vi "1midterm.vi"() -> ()   [LabVIEW 2024]
uses:
  <userlib>/SerialVIs/subs/portX.xctl
panel:
  in  "File Path 5":path=path "C:/Users/mbyjo/Downloads/tish---success!-made-with-Voicemod.wav"
  in  "File Path 4":path=path "C:/Users/mbyjo/Downloads/eye-of-the-tiger-intro-made-with-Voicemod.wav"
  in  "File Path 3":path=path "C:/Users/mbyjo/Downloads/game-over-made-with-Voicemod.wav"
  in  "File Path 2":path=path "C:/Users/mbyjo/Downloads/evil-laugh-made-with-Voicemod.wav"
  in  "File Path":path=path "C:/Users/mbyjo/Downloads/saw-do-you-wanna-play-a-game_-made-with-Voicemod.wav"
  out "Arm Range 2":cluster{"X":dbl, "Y":dbl}[](graph)
  out "Angle 3":dbl
  out "Angle 2":dbl
  out "Angle1":dbl
  out "Arm Range 1":picture
  out "Robot arm Final Position":cluster{"x2":dbl, "y2":dbl}
  out "2D Simulation of Robot Arm":picture
  out "Angles(q)":dbl[](array[numeric])
  in  "Arm Lengths":cluster{"L 1":dbl, "L 2":dbl, "L4":dbl}
  in  "portX":refnum<visa-resource-name>(xcontrol)
  # "DO YOU WANNA PLAY A GAME?"
  # "PRESS THE ARROW TO GET STARTED!"
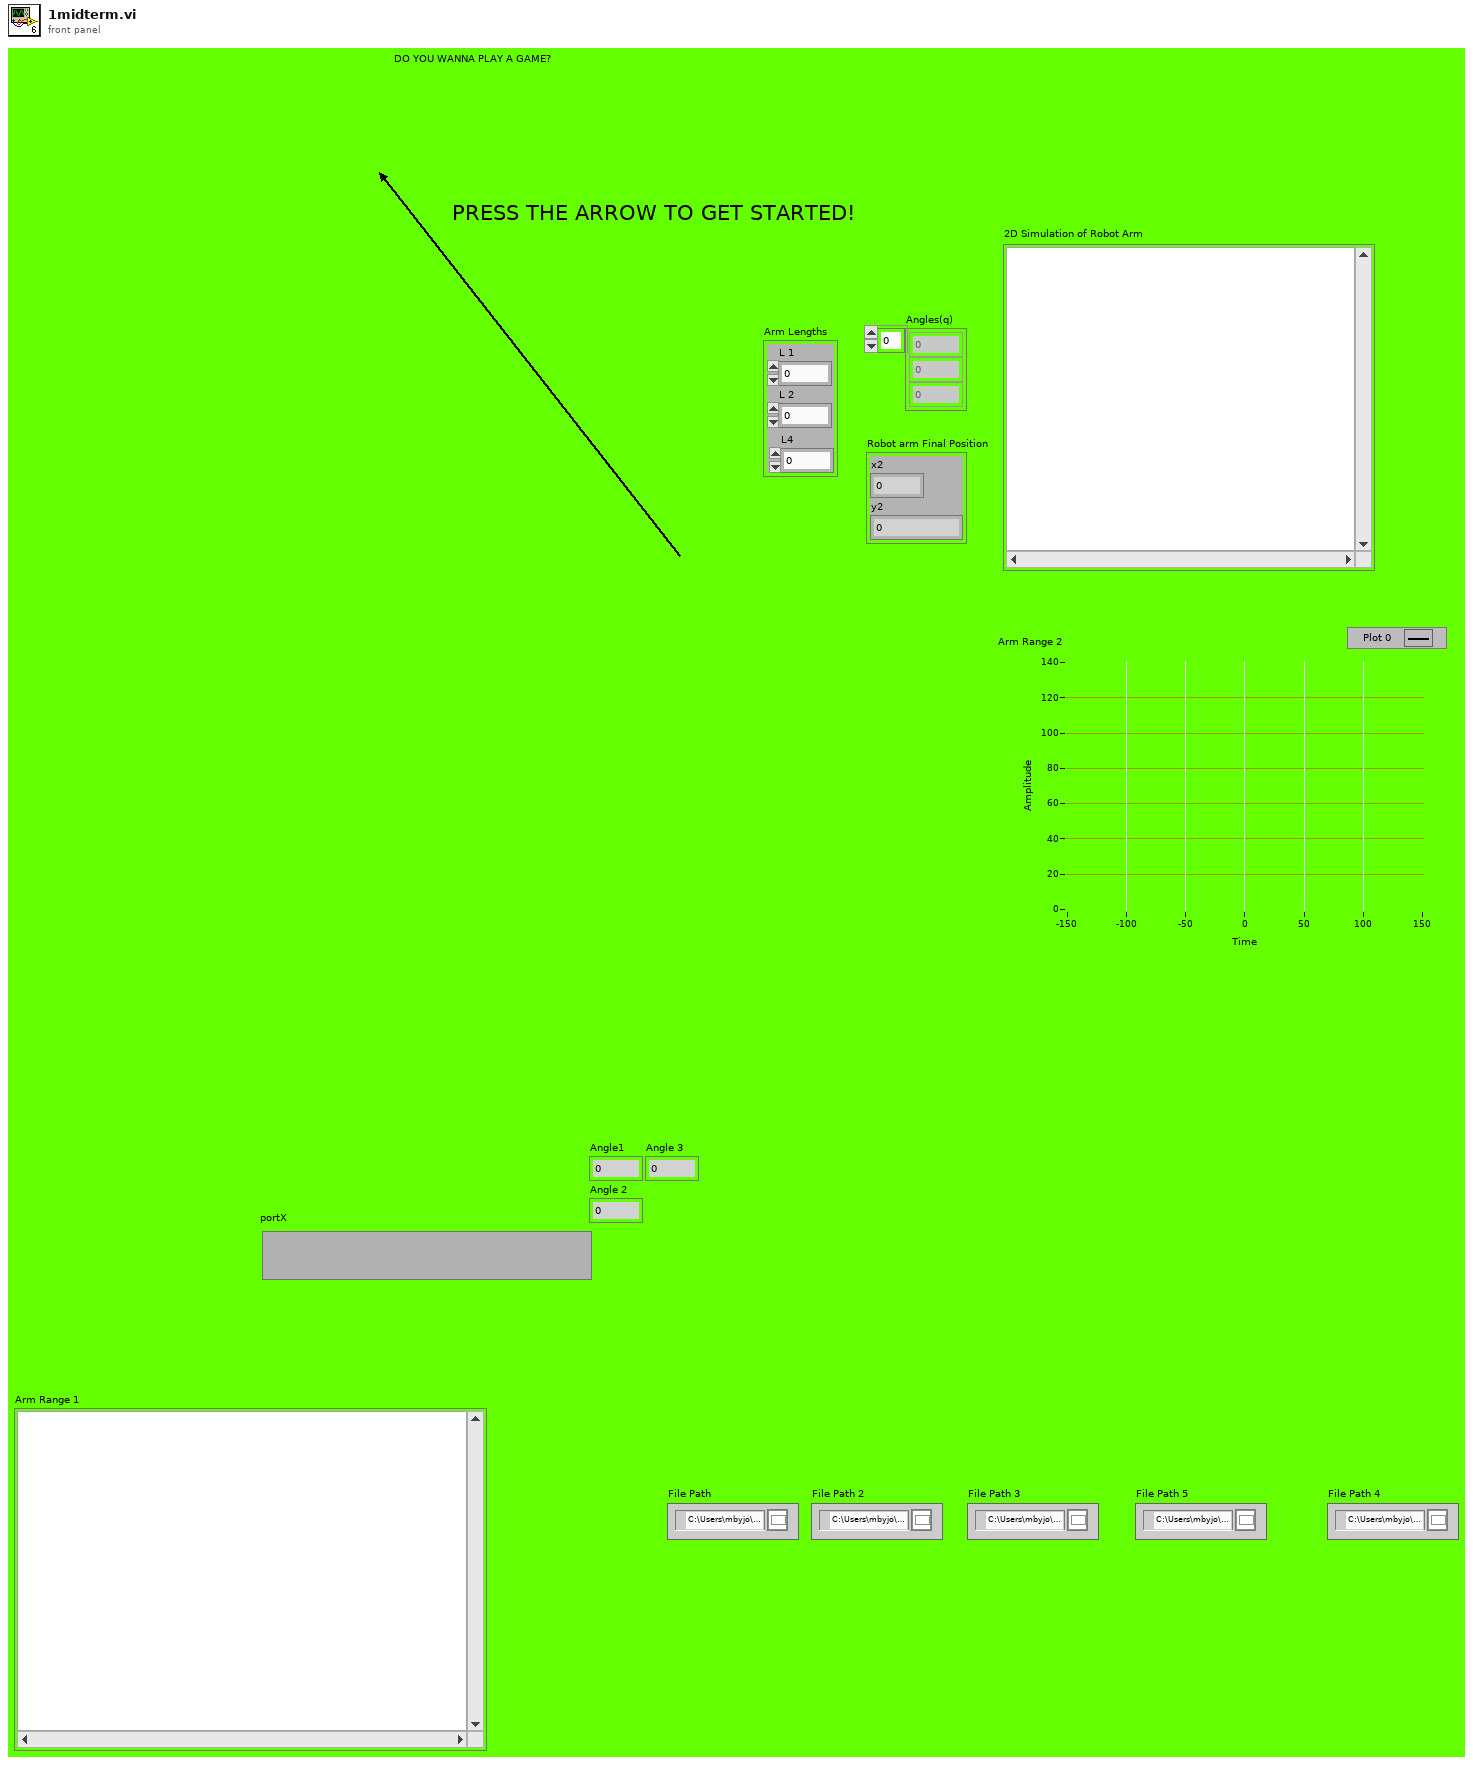
[diagram p1: front panel]
types:
  T1 = cluster{"Width":u16, "Style":enum32{"Solid", "Dash", "Dot", "DashDot", "DashDotDot"}}
  T2 = cluster{"Angles(q)[0]":dbl, "Angles(q)[1]":dbl, "Angles(q)[2]":dbl, "Angles(q)[3]":dbl, "Angles(q)[4]":dbl, "Angles(q)[5]":dbl, "Angles(q)[6]":dbl, "Angles(q)[7]":dbl, "Angles(q)[8]":dbl}
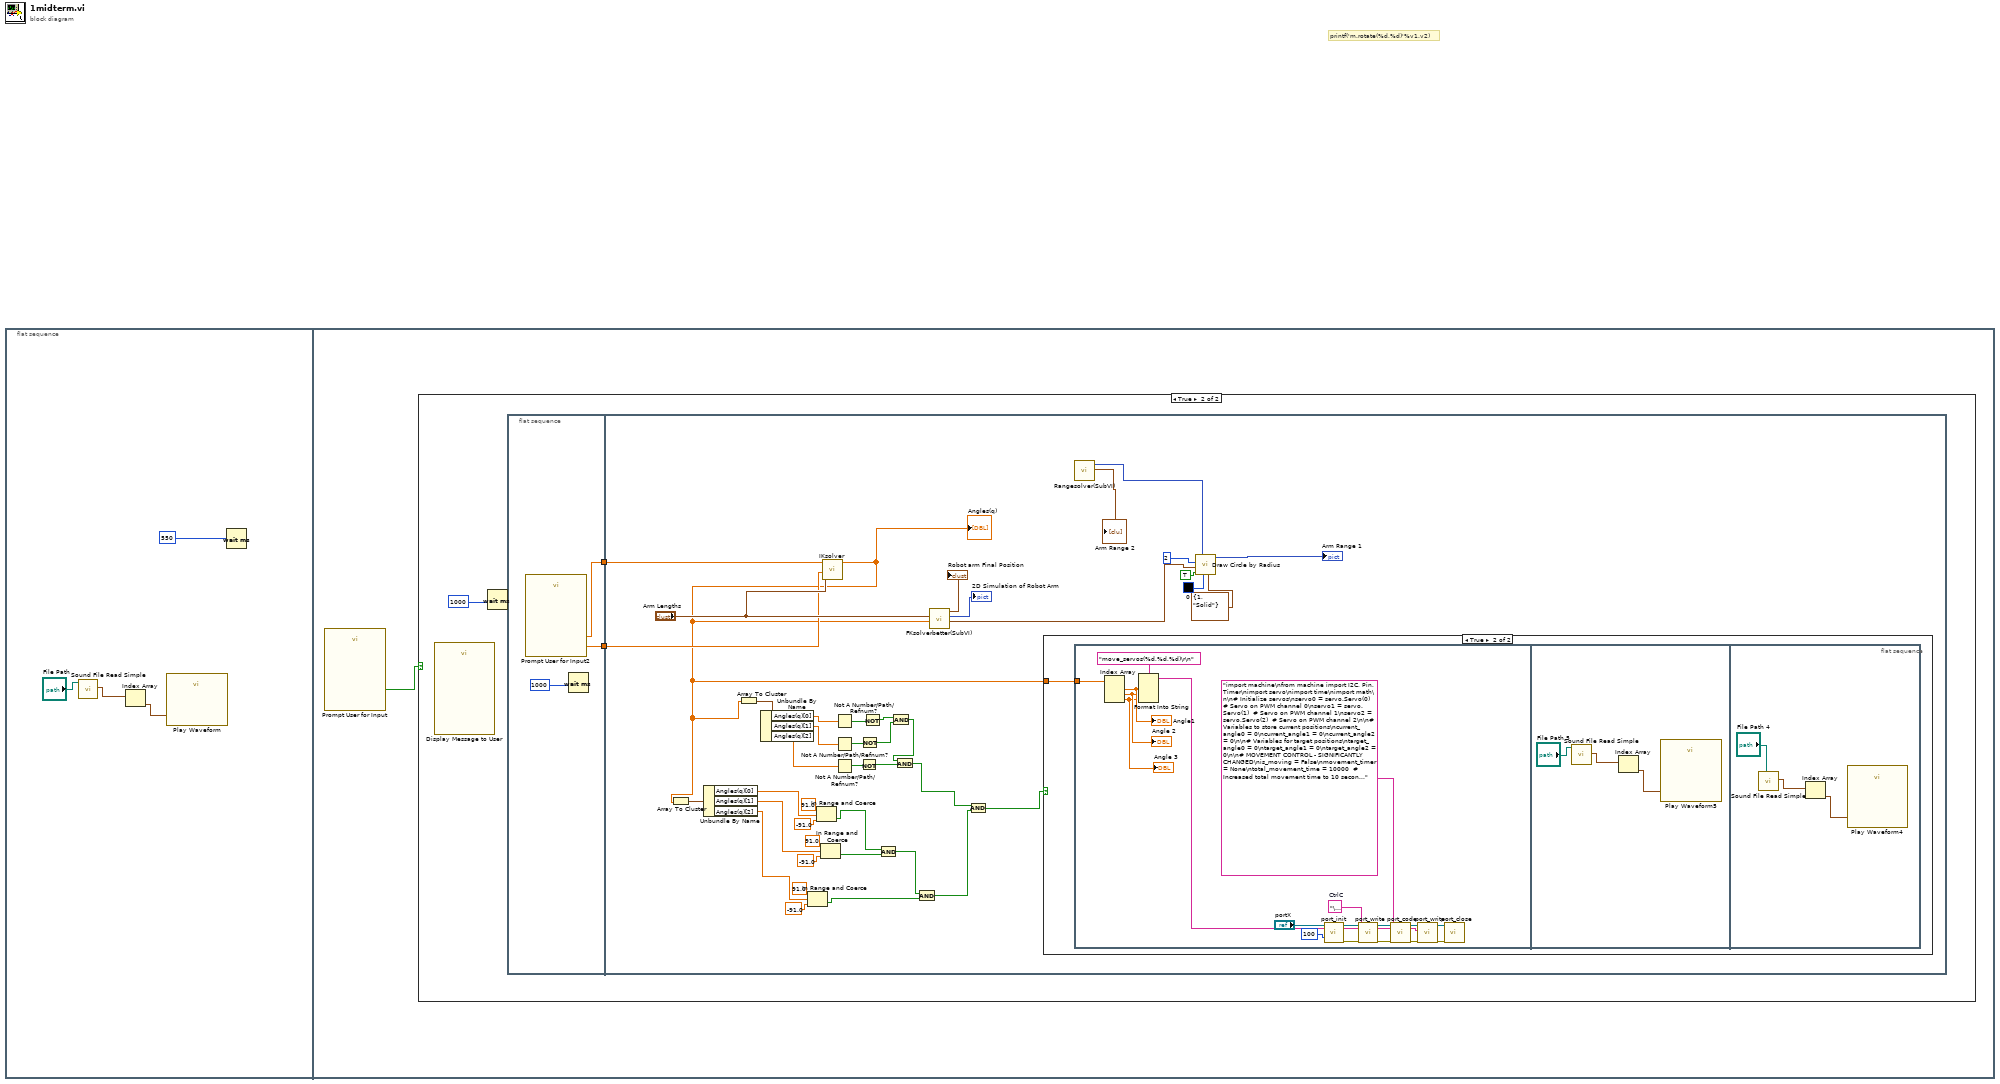
[diagram p0: block diagram]
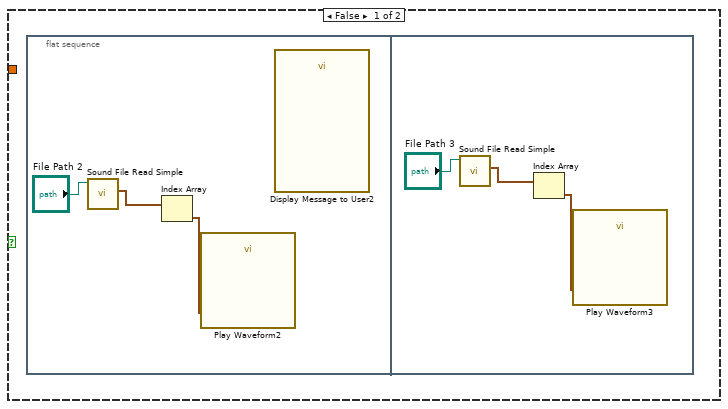
[diagram p3: hidden frame]
diagram:
  # "printf('m.rotate(%d,%d)'%v1.v2)"
  n1 = flat-sequence {
    frame #0 {
      n2 = call <vilib>:"Sound File Read Simple.vi"("path"="File Path") -> ("data"=w3:waveform(dbl)[])  [unwired: 7 in, 3 out]
      n3 = Index Array(array=w3) -> (element=w4:waveform(dbl))  [unwired: 1 in]
      n4 = call "Play Waveform"("Data"=w4) -> ()  [unwired: 18 in, 1 out]
      n5 = Wait (ms)(milliseconds to wait=u32 550) -> ()  [unwired: 1 out]
    }
    frame #1 {
      n6 = call "Prompt User for Input"() -> ("YES"=w5:bool)  [unwired: 16 in, 3 out]
      n7 = case shown="True" w5 {
        frame False {
        }
        frame True {
          n8 = call "Display Message to User"() -> ()  [unwired: 10 in, 2 out]
          n9 = Wait (ms)(milliseconds to wait=u32 1000) -> ()  [unwired: 1 out]
          n10 = flat-sequence {
            tunnel: [w10] -> w7
            tunnel: [w9] -> w6
            tunnel: w7 -> [w42]
            tunnel: w6 -> [w41]
            frame #0 {
              n11 = call "Prompt User for Input2"() -> ("y"=w10:dbl, "x"=w9:dbl)  [unwired: 16 in, 2 out]
              n12 = Wait (ms)(milliseconds to wait=u32 1000) -> ()  [unwired: 1 out]
            }
            frame #1 {
              n13 = call "IKsolver.vi"("y"=w42, "Arm Lengths"="Arm Lengths", "x"=w41) -> ("Angles(q)"=w29:dbl[])  [unwired: 8 in]
              "Angles(q)" <- w29
              n14 = Array To Cluster(array=w29) -> (cluster=w28:T2)
              n15 = Unbundle By Name(w28) -> ("Angles(q)[0]"=w26:dbl, "Angles(q)[1]"=w18:dbl, "Angles(q)[2]"=w17:dbl)
              n16 = Array To Cluster(array=w29) -> (cluster=w40:T2)
              n17 = Unbundle By Name(w40) -> ("Angles(q)[0]"=w39:dbl, "Angles(q)[1]"=w38:dbl, "Angles(q)[2]"=w37:dbl)
              n18 = In Range and Coerce(upper limit=91.0, x=w17, lower limit=-91.0) -> (In Range?=w13:bool)  [unwired: 1 out]
              n19 = In Range and Coerce(upper limit=91.0, x=w26, lower limit=-91.0) -> (In Range?=w15:bool)  [unwired: 1 out]
              n20 = In Range and Coerce(upper limit=91.0, x=w18, lower limit=-91.0) -> (In Range?=w16:bool)  [unwired: 1 out]
              n21 = Not A Number/Path/Refnum?(number/path/refnum=w38) -> (NaN/Path/Refnum?=w35:bool)
              n22 = Not A Number/Path/Refnum?(number/path/refnum=w39) -> (NaN/Path/Refnum?=w36:bool)
              n23 = Not A Number/Path/Refnum?(number/path/refnum=w37) -> (NaN/Path/Refnum?=w34:bool)
              n24 = Not(x=w34) -> (.not. x?=w31:bool)
              n25 = Not(x=w35) -> (.not. x?=w32:bool)
              n26 = Not(x=w36) -> (.not. x?=w33:bool)
              n27 = And(x=w15, y=w16) -> (x .and. y?=w14:bool)
              n28 = And(x=w33, y=w32) -> (x .and. y?=w30:bool)
              n29 = And(x=w30, y=w31) -> (x .and. y?=w24:bool)
              n30 = And(x=w14, y=w13) -> (x .and. y?=w12:bool)
              n31 = call "FKsolverbetter(SubVI).vi"("q"=w29, "Arm Lengths"="Arm Lengths") -> ("end (2D)"=w51:cluster{"x":dbl, "y":dbl}, "2D Picture 2"=→"2D Simulation of Robot Arm":picture, "Robot arm Final Position"=→"Robot arm Final Position":cluster{"x2":dbl, "y2":dbl})  [unwired: 6 in]
              n32 = And(x=w24, y=w12) -> (x .and. y?=w23:bool)
              n33 = case shown="True" w23 {
                tunnel: w29 -> [_ w60]
                frame False {
                  n34 = flat-sequence {
                    frame #0 {
                      n35 = call <vilib>:"Sound File Read Simple.vi"("path"="File Path 2") -> ("data"=w55:waveform(dbl)[])  [unwired: 7 in, 3 out]
                      n36 = Index Array(array=w55) -> (element=w56:waveform(dbl))  [unwired: 1 in]
                      n37 = call "Play Waveform2"("Data"=w56) -> ()  [unwired: 18 in, 1 out]
                      n38 = call "Display Message to User2"() -> ()  [unwired: 10 in, 2 out]
                    }
                    frame #1 {
                      n39 = call <vilib>:"Sound File Read Simple.vi"("path"="File Path 3") -> ("data"=w58:waveform(dbl)[])  [unwired: 7 in, 3 out]
                      n40 = Index Array(array=w58) -> (element=w59:waveform(dbl))  [unwired: 1 in]
                      n41 = call "Play Waveform3"("Data"=w59) -> ()  [unwired: 18 in, 1 out]
                    }
                  }
                }
                frame True {
                  n42 = flat-sequence {
                    tunnel: w60 -> [w61]
                    frame #0 {
                      w62 = "\u0003"  # CtrlC
                      n43 = Index Array(array=w61) -> (element #1=w75:dbl, element #2=w74:dbl, element #3=w73:dbl)  [unwired: 3 in]
                      "Angle1" <- w75
                      "Angle 2" <- w74
                      "Angle 3" <- w73
                      n44 = Format Into String(format string="move_servos(%d,%d,%d)\r\n", w75, w74, w73) -> (resulting string=w76:string)  [unwired: 2 in, 1 out]
                      n45 = call <userlib>:"port_init.vi"("Timeout (ms)"=u32 100, "VISA Refnum in"="portX") -> ("error out"=w67:errorcluster, "VISA Refnum out"=w66:refnum<visa-resource-name>)  [unwired: 8 in]
                      n46 = call <userlib>:"port_write.vi"("error in (no error)"=w67, "write buffer"=w62, "VISA Refnum in"=w66) -> ("error out"=w69:errorcluster, "VISA Refnum out"=w70:refnum<visa-resource-name>)  [unwired: 7 in]
                      n47 = call <userlib>:"port_code.vi"("error in (no error)"=w69, "Code to run"="import machine\nfrom machine import I2C, Pin, Timer\nimport servo\nimport time\nimport math\n\n# Initialize servos\nservo0 = servo.Servo(0)  # Servo on PWM channel 0\nservo1 = servo.Servo(1)  # Servo on PWM channel 1\nservo2 = servo.Servo(2)  # Servo on PWM channel 2\n\n# Variables to store current positions\ncurrent_angle0 = 0\ncurrent_angle1 = 0\ncurrent_angle2 = 0\n\n# Variables for target positions\ntarget_angle0 = 0\ntarget_angle1 = 0\ntarget_angle2 = 0\n\n# MOVEMENT CONTROL - SIGNIFICANTLY CHANGED\nis_moving = False\nmovement_timer = None\ntotal_movement_time = 10000  # Increased total movement time to 10 seconds for slower movement\nupdate_interval = 20  # Reduced update interval to 20ms for smoother motion\nmovement_steps = 0  # Will be calculated based on largest angle change\ncurrent_step = 0    # Track which step we're on\n\ndef move_servos(angle0, angle1, angle2):\n    \"\"\"\n    Immediately move servos to specified angles.\n    \"\"\"\n    servo0.write(angle0)\n    servo1.write(angle1)\n    servo2.write(angle2)\n\ndef timer_callback(timer):\n    \"\"\"\n    This function is called by the timer at regular intervals.\n    It moves the servos gradually along a predetermined path.\n    \"\"\"\n    global current_angle0, current_angle1, current_angle2, is_moving, current_step\n    \n    # Check if we've completed all steps\n    if current_step >= movement_steps:\n        # We've reached the target, stop moving\n        is_moving = False\n        timer.deinit()  # Stop the timer\n        \n        # Set exact target angles\n        move_servos(target_angle0, target_angle1, target_angle2)\n        current_angle0 = target_angle0\n        current_angle1 = target_angle1\n        current_angle2 = target_angle2\n        print(\"Movement complete.\")\n        return\n    \n    # Calculate new intermediate positions based on linear interpolation\n    fraction = (current_step + 1) / movement_steps\n    \n    # Compute new angles based on the step\n    new_angle0 = start_angle0 + (target_angle0 - start_angle0) * fraction\n    new_angle1 = start_angle1 + (target_angle1 - start_angle1) * fraction\n    new_angle2 = start_angle2 + (target_angle2 - start_angle2) * fraction\n    \n    # Move servos to new positions\n    move_servos(new_angle0, new_angle1, new_angle2)\n    \n    # Update current angles\n    current_angle0 = new_angle0\n    current_angle1 = new_angle1\n    current_angle2 = new_angle2\n    \n    # Increment step\n    current_step += 1\n\ndef start_slow_movement(new_angle0, new_angle1, new_angle2):\n    \"\"\"\n    Start slow movement to new target angles.\n    Uses linear interpolation over fixed time period.\n    \"\"\"\n    global target_angle0, target_angle1, target_angle2, is_moving, movement_timer\n    global start_angle0, start_angle1, start_angle2, movement_steps, current_step\n    \n    # Store starting positions\n    start_angle0 = current_angle0\n    start_angle1 = current_angle1\n    start_angle2 = current_angle2\n    \n    # Set new targets\n    target_angle0 = new_angle0\n    target_angle1 = new_angle1\n    target_angle2 = new_angle2\n    \n    # Calculate number of steps based on desired time and update interval\n    movement_steps = int(total_movement_time / update_interval)\n    current_step = 0\n    \n    print(f\"Starting {total_movement_time/1000:.1f}-second movement to: {new_angle0:.1f}, {new_angle1:.1f}, {new_angle2:.1f}\")\n    print(f\"Movement will take exactly {total_movement_time/1000:.1f} seconds\")\n    print(f\"Using {movement_steps} steps with {update_interval}ms interval\")\n    \n    # If already moving, stop the current movement\n    if is_moving and movement_timer is not None:\n        movement_timer.deinit()\n    \n    # Start new movement\n    is_moving = True\n    movement_timer = Timer(-1)  # Use any available timer\n    movement_timer.init(period=update_interval, mode=Timer.PERIODIC, callback=timer_callback)\n\ndef move_to_position(x, y, link1_length, link2_length):\n    \"\"\"\n    Move the robot arm to a position (x,y) using inverse kinematics.\n    Uses timer for slow, controlled movement over exactly 10 seconds.\n    \n    Parameters:\n    - x, y: Target position coordinates\n    - link1_length, link2_length: Lengths of the two arm links\n    \n    Returns:\n    - True if the position is reachable, False otherwise\n    \"\"\"\n    import math\n    \n    # Check if position is within reach\n    distance = math.sqrt(x**2 + y**2)\n    if distance > (link1_length + link2_length) or distance < abs(link1_length - link2_length):\n        print(\"Position out of reach\")\n        return False\n    \n    # Calculate angles using inverse kinematics\n    cos_angle2 = (x**2 + y**2 - link1_length**2 - link2_length**2) / (2 * link1_length * link2_length)\n    if cos_angle2 > 1 or cos_angle2 < -1:\n        print(\"Position out of reach (trigonometric error)\")\n        return False\n        \n    angle2 = math.acos(cos_angle2)  # Elbow angle\n    \n    # Convert to degrees for servo control\n    angle2_deg = math.degrees(angle2)\n    \n    # Calculate first joint angle\n    k1 = link1_length + link2_length * cos_angle2\n    k2 = link2_length * math.sin(angle2)\n    angle1 = math.atan2(y, x) - math.atan2(k2, k1)\n    angle1_deg = math.degrees(angle1)\n    \n    # Calculate third angle to keep chair upright\n    angle3_deg = -(angle1_deg + angle2_deg)\n    \n    # Start exactly 10-second movement to target\n    start_slow_movement(angle1_deg, angle2_deg, angle3_deg)\n    \n    return True\n\n# Initialize by setting servos to starting position\nmove_servos(0, 0, 0)\ncurrent_angle0 = 0\ncurrent_angle1 = 0\ncurrent_angle2 = 0\n\n# Example usage:\n# To move to a position (x=10, y=5) with arm links of lengths 10 and 8\n# move_to_position(10, 5, 10, 8)", "VISA Refnum in"=w70) -> ("error out"=w78:errorcluster, "VISA Refnum out"=w77:refnum<visa-resource-name>)  [unwired: 7 in]
                      n48 = call <userlib>:"port_write.vi"("error in (no error)"=w78, "write buffer"=w76, "VISA Refnum in"=w77) -> ("error out"=w72:errorcluster, "VISA Refnum out"=w71:refnum<visa-resource-name>)  [unwired: 7 in]
                      n49 = call <userlib>:"port_close.vi"("error in (no error)"=w72, "VISA Refnum in"=w71) -> ()  [unwired: 10 in]
                    }
                    frame #1 {
                      n50 = call <vilib>:"Sound File Read Simple.vi"("path"="File Path 5") -> ("data"=w80:waveform(dbl)[])  [unwired: 7 in, 3 out]
                      n51 = Index Array(array=w80) -> (element=w81:waveform(dbl))  [unwired: 1 in]
                      n52 = call "Play Waveform5"("Data"=w81) -> ()  [unwired: 18 in, 1 out]
                    }
                    frame #2 {
                      n53 = call <vilib>:"Sound File Read Simple.vi"("path"="File Path 4") -> ("data"=w83:waveform(dbl)[])  [unwired: 7 in, 3 out]
                      n54 = Index Array(array=w83) -> (element=w84:waveform(dbl))  [unwired: 1 in]
                      n55 = call "Play Waveform4"("Data"=w84) -> ()  [unwired: 18 in, 1 out]
                    }
                  }
                }
              }
              n56 = call "Rangesolver(SubVI).vi"() -> ("XY Graph"=→"Arm Range 2":cluster{"X":dbl, "Y":dbl}[], "new picture"=w48:picture)  [unwired: 10 in]
              n57 = call <vilib>:"Draw Circle by Radius.vi"("pen"=T1 {"Width"=1, "Style"=enum."Solid"}, "color(black)"=u32 0, "fill?(F)"=TRUE, "pixel center"=w51, "radius"=i16 2, "picture"=w48) -> ("new picture"=→"Arm Range 1":picture)  [unwired: 5 in]
            }
          }
        }
      }
    }
  }
